vi "Next Search ID Number.vi"() -> (3 "Next ID #":i32)   [LabVIEW 2020, in "Better Search.lvlib" / "Search.lvclass"]
uses:
  Search.lvclass
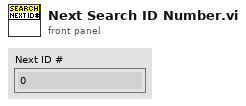
[diagram p1: front panel]
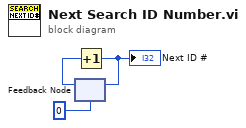
[diagram p0: block diagram]
diagram:
  n1 = feedback #1(0) -> (w2:i32)
  n2 = Increment(x=w2) -> (x+1=w3:i32)
  "Next ID #" <- w3
  n3 = feedback-in #1(w3) -> ()
